vi "Organise_Movies.vi"() -> ()   [LabVIEW 2011]
uses:
  Anemometry Sub Vis/Globals/Constants_global.vi
panel:
  out "appended path":path
  out "Filename":string
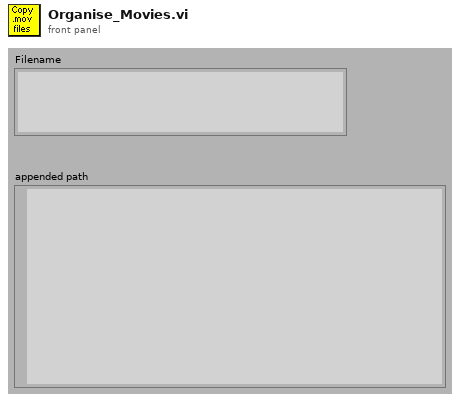
[diagram p1: front panel]
types:
  T1 = cluster{"second":i32, "minute":i32, "hour":i32, "day of month":i32, "month":i32, "year":i32, "day of week":i32, "day of year":i32, "is DST":i32}
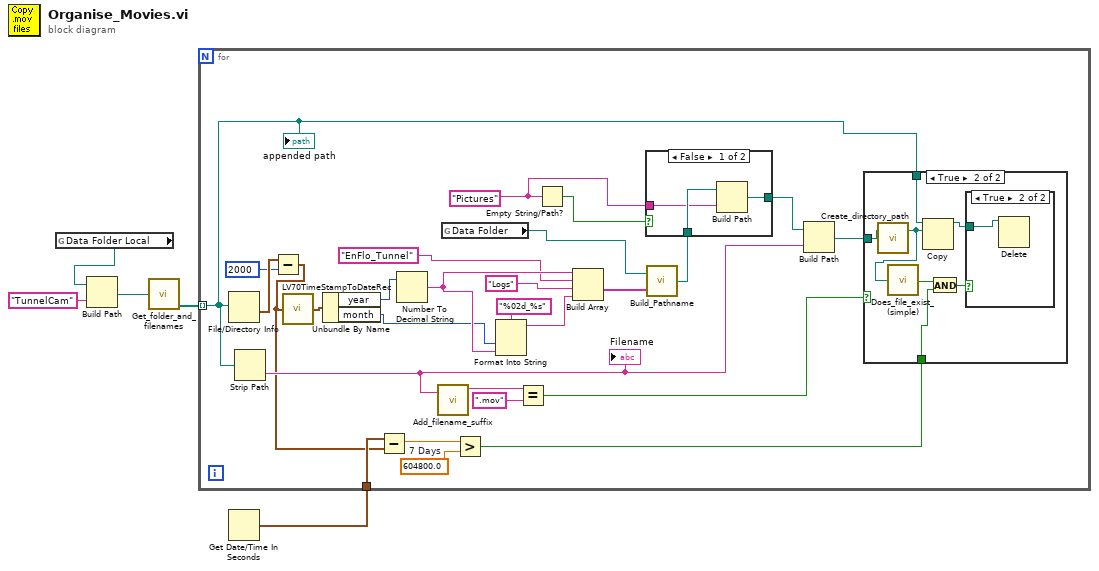
[diagram p0: block diagram]
diagram:
  n1 = global read "Constants_global.vi" "Data Folder Local"() -> (w4:path)
  n2 = Build Path(base path=w4, name or relative path="TunnelCam") -> (appended path=w3:path)
  n3 = call "Get_folder_and_filenames.vi"("file path (dialog if empty)"=w3) -> ("Files"=w5:path[])  [unwired: 1 out]
  n4 = Get Date/Time In Seconds() -> (seconds since 1Jan1904=w1:timestamp)
  n5 = for {
    tunnel: w5 -> [w18] mode=indexing
    tunnel: w1 -> [w12]
    w10 = 604800.0  # 7 Days
    w20 = "Pictures" ("Log Folder")
    n6 = File/Directory Info(path=w18) -> (last mod=w8:timestamp)  [unwired: 1 in, 6 out]
    n7 = Strip Path(path=w18) -> (name=w16:string)  [unwired: 1 out]
    "Filename" <- w16
    n8 = Subtract(x=w8, y=2000) -> (x-y=w6:timestamp)
    n9 = call <vilib>:"LV70TimeStampToDateRec.vi"("time stamp"=w6) -> ("date time rec"=w23:T1)
    n10 = Unbundle By Name(w23) -> ("year"=w24:i32, "month"=w28:i32)
    n11 = Subtract(x=w12, y=w6) -> (x-y=w11:dbl)
    n12 = Number To Decimal String(number=w24) -> (decimal integer string=w29:string)  [unwired: 1 out]
    n13 = call "Add_filename_suffix.vi"("Filename"=w16) -> ("Original Suffix"=w15:string)  [unwired: 1 in, 3 out]
    n14 = global read "Constants_global.vi" "Data Folder"() -> (w21:path)
    n15 = Greater?(x=w11, y=w10) -> (0:w9:bool)
    n16 = Format Into String(format string="%02d_%s", w28, w29) -> (resulting string=w31:string)  [unwired: 2 in, 1 out]
    n17 = Equal?(x=w15, y=".mov") -> (x = y?=w13:bool)
    n18 = Empty String/Path?(string/path=w20) -> (empty?=w26:bool)
    n19 = Build Array(w29, "EnFlo_Tunnel" ("Rig Setup"), "Logs", w31) -> (w32:string[])
    n20 = call "Build_Pathname.vi"("Output Array"=w32, "Pathname"=w21) -> ("Appended path"=w25:path)
    n21 = case shown="False" w26 {
      tunnel: w25 -> [w43 w44]
      tunnel: [w42 w44] -> w22
      tunnel: w20 -> [w41 _]
      frame False {
        n22 = Build Path(base path=w43, name or relative path=w41) -> (appended path=w42:path)
      }
      frame True {
      }
    }
    n23 = Build Path(base path=w22, name or relative path=w16) -> (appended path=w17:path)
    n24 = case shown="True" w13 {
      tunnel: w18 -> [_ w38]
      tunnel: w17 -> [_ w39]
      tunnel: w9 -> [_ w33]
      frame False {
      }
      frame True {
        n25 = call "Create_directory_path.vi"("Path name"=w39) -> ("Path name Out"=w35:path)  [unwired: 1 in, 1 out]
        n26 = call "Does_file_exist_(simple).vi"("Pathname"=w35) -> ("exists?"=w34:bool)
        n27 = Copy(10:w35, 11:w38) -> (3:w37:path)  [unwired: 1 in, 4 out]
        n28 = And(x=w34, y=w33) -> (x .and. y?=w36:bool)
        n29 = case shown="True" w36 {
          tunnel: w37 -> [_ w40]
          frame False {
          }
          frame True {
            n30 = Delete(path (use dialog)=w40) -> ()  [unwired: 1 in, 6 out]
          }
        }
      }
    }
    "appended path" <- w18
  }
